vi "testPlayer.vi"() -> ()   [LabVIEW 2019]
uses:
  Player.lvclass/Player.ctl
  Player.lvclass
panel:
  out "userName":string
  out "highScore":u64
  out "Current Score":i32
  out "High Score Updated?":bool
  in  "User Namer":string
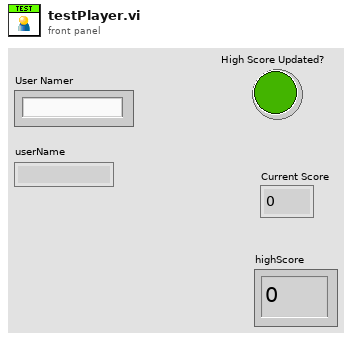
[diagram p1: front panel]
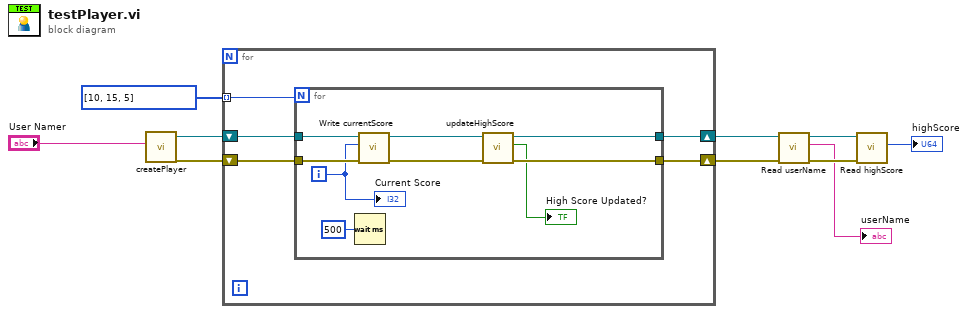
[diagram p0: block diagram]
diagram:
  n1 = call "createPlayer.vi"("Name"="User Namer") -> ("error out"=w8:errorcluster, "Player out"=w9:refnum<class "Player.lvclass">)  [unwired: 9 in]
  n2 = for {
    shift-right: [w13] -> w7
    shift-left: w9 -> [w15]
    shift-right: [w12] -> w6
    shift-left: w8 -> [w14]
    tunnel: i32[] [10, 15, 5] -> [w11] mode=indexing
    n3 = for {
      N: w11 -> [_]
      tunnel: w15 -> [w24]
      tunnel: w14 -> [w23]
      tunnel: [w19] -> w13
      tunnel: [w21] -> w12
      i -> [w16]
      n4 = Wait (ms)(milliseconds to wait=u32 500) -> ()  [unwired: 1 out]
      n5 = call "Write currentScore.vi"("error in (no error)"=w23, "currentScore"=w16, "Player in"=w24) -> ("error out"=w22:errorcluster, "Player out"=w20:refnum<class "Player.lvclass">)  [unwired: 7 in]
      n6 = call "updateHighScore.vi"("error in (no error)"=w22, "Player in"=w20) -> ("error out"=w21:errorcluster, "High Score Updated?"=→"High Score Updated?":bool, "Player out"=w19:refnum<class "Player.lvclass">)  [unwired: 7 in]
      "Current Score" <- w16
    }
  }
  n7 = call "Read userName.vi"("error in (no error)"=w6, "Player in"=w7) -> ("error out"=w4:errorcluster, "userName"=→"userName":string, "Player out"=w5:refnum<class "Player.lvclass">)  [unwired: 7 in]
  n8 = call "Read highScore.vi"("error in (no error)"=w4, "Player in"=w5) -> ("highScore"=→"highScore":u64)  [unwired: 7 in, 2 out]
